vi "FTW-Regex-Replacements.vi"(0 "String":string, 5 "Value Replacements":T1(array[cluster]), 11 "error in":errorcluster) -> (4 "String out":string, 6 "Number of Replacements":i32[](array[numeric]), 15 "error out":errorcluster)   [LabVIEW 2015]
panel:
  # "Inputs"
  # "Outputs"
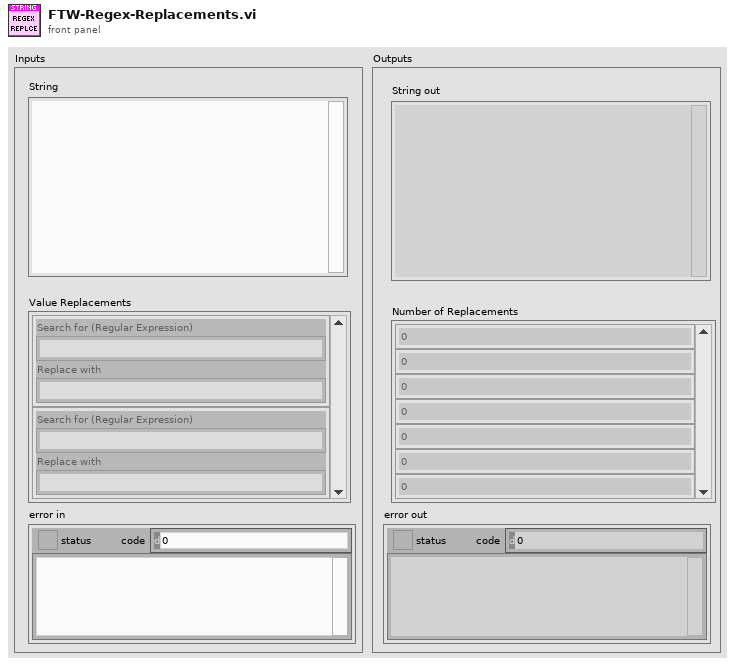
[diagram p1: front panel]
types:
  T1 = cluster{"Search for (Regular Expression)":string, "Replace with":string}[]
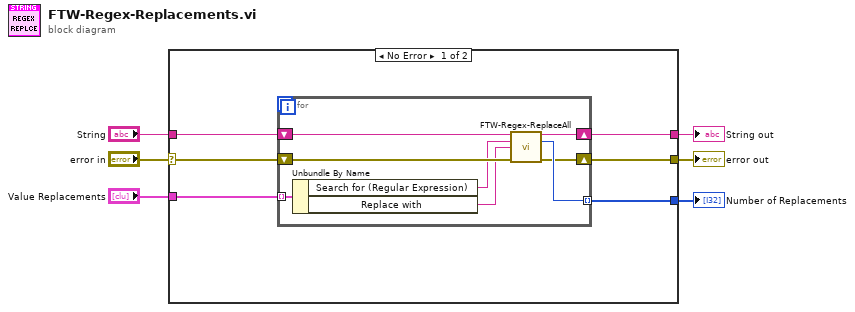
[diagram p0: block diagram]
diagram:
  n1 = case shown="No Error" "error in" {
    selector: "error in" -> [w11 w21]
    tunnel: [w8 w21] -> w6
    tunnel: "String" -> [w12 _]
    tunnel: [w9 _] -> w2
    tunnel: "Value Replacements" -> [w10 _]
    tunnel: [w7 _] -> w1
    frame No Error {
      n2 = for {
        shift-right: [w18] -> w9
        shift-left: w12 -> [w19]
        tunnel: w10 -> [w20] mode=indexing
        shift-right: [w16] -> w8
        shift-left: w11 -> [w15]
        tunnel: [w17] -> w7 mode=indexing
        n3 = Unbundle By Name(w20) -> ("Search for (Regular Expression)"=w13:string, "Replace with"=w14:string)
        n4 = call "FTW-Regex-ReplaceAll.vi"("String"=w19, "Search for (Regular Expression)"=w13, "Replace with"=w14, "error in"=w15) -> ("String out"=w18:string, "Number of Replacements"=w17:i32, "error out"=w16:errorcluster)  [unwired: 9 in]
      }
    }
    frame Error {
    }
  }
  "error out" <- w6
  "String out" <- w2
  "Number of Replacements" <- w1
